vi "循环语句.vi"() -> ()   [LabVIEW 2018]
uses:
  <vilib>/measure/maspectr.llb/FFT Power Spectrum and PSD for 1 Chan.vi
  <vilib>/measure/NI_MABase.lvlib
  <vilib>/measure/NI_MAPro.lvlib
panel:
  in  "停止":bool
  out "频谱":cluster{"f0":dbl, "df":dbl, "magnitude":dbl[]}(graph)
  out "信号":waveform(dbl)[](graph)
  in  "采样率":dbl(ring) items=["100000000", "1000000", "50000000"]
  in  "频率":dbl(knob) scale=0.0..50000000.0 scale format="%#_6p"
  in  "枚举":enum16{"正弦波", "方波"}(ring)
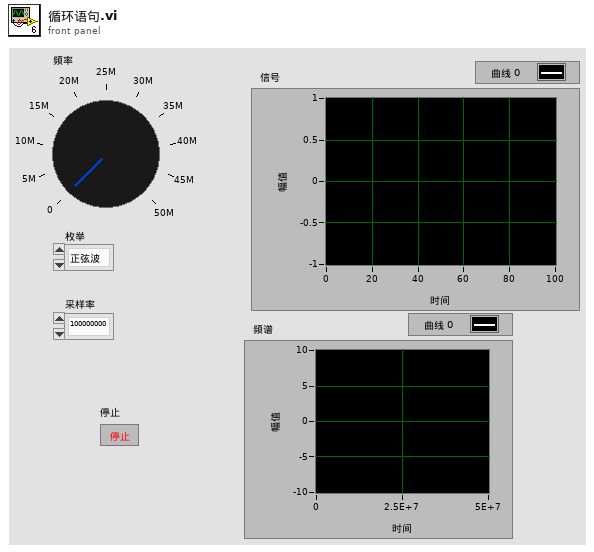
[diagram p1: front panel]
types:
  T1 = cluster{"averaging mode":enum16{"No averaging", "Vector averaging", "RMS averaging", "Peak hold"}, "weighting mode":enum16{"Linear", "Exponential"}, "number of averages":u32}
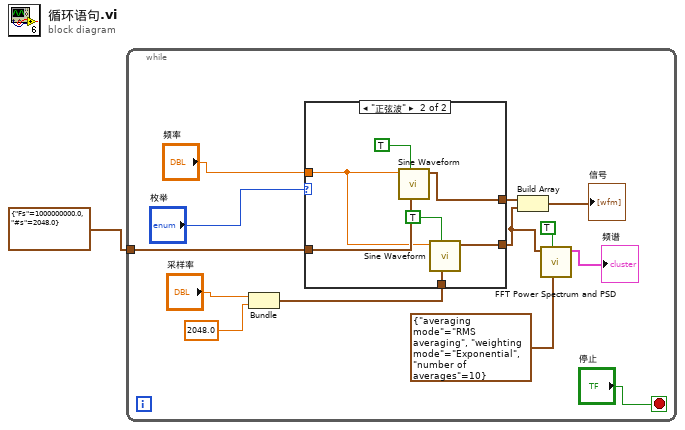
[diagram p0: block diagram]
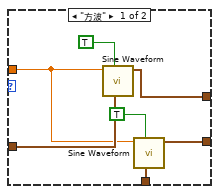
[diagram p2: hidden frame]
diagram:
  n1 = while {
    tunnel: cluster{"Fs":dbl, "#s":dbl} {"Fs"=1000000000.0, "#s"=2048.0} ("sampling info") -> [w12]
    stop <- "停止" stop-if-true
    n2 = Bundle("采样率"="采样率", 2048.0) -> (w9:cluster{"采样率":dbl, dbl})  [unwired: 1 in]
    n3 = case shown="\"正弦波\"" "枚举" {
      tunnel: "频率" -> [w20 w27]
      tunnel: w12 -> [w21 w28]
      tunnel: w9 -> [w19 w26]
      tunnel: [w16 w23] -> w8
      tunnel: [w15 w22] -> w6
      frame "方波" {
        n4 = call <vilib>:"Sine Waveform.vi"("sampling info"=w21, "reset signal"=TRUE, "frequency"=w20) -> ("signal out"=w16:waveform(dbl))  [unwired: 7 in, 1 out]
        n5 = call <vilib>:"Sine Waveform.vi"("sampling info"=w19, "reset signal"=TRUE, "frequency"=w20) -> ("signal out"=w15:waveform(dbl))  [unwired: 7 in, 1 out]
      }
      frame "正弦波" {
        n6 = call <vilib>:"Sine Waveform.vi"("sampling info"=w28, "reset signal"=TRUE, "frequency"=w27) -> ("signal out"=w23:waveform(dbl))  [unwired: 7 in, 1 out]
        n7 = call <vilib>:"Sine Waveform.vi"("sampling info"=w26, "reset signal"=TRUE, "frequency"=w27) -> ("signal out"=w22:waveform(dbl))  [unwired: 7 in, 1 out]
      }
    }
    n8 = Build Array(w8, w6) -> (→"信号":waveform(dbl)[])
    n9 = call-poly <vilib>:"FFT Power Spectrum and PSD.vi"("averaging parameters"=T1 {"averaging mode"=enum."RMS averaging", "weighting mode"=enum."Exponential", "number of averages"=10}, "restart averaging (F)"=TRUE, "time signal"=w6) -> ("Power Spectrum / PSD"=→"频谱":cluster{"f0":dbl, "df":dbl, "magnitude":dbl[]})  [unwired: 5 in, 3 out]
  }
